vi "LinearIndicatorMarker.vi"(4 "Marker Height":i32, 5 "Group":string, 6 "Value":dbl, 7 "Color":u32(colorbox)=6618880, 10 "RectangleSizeAndLocation":T2, 11 "Image":T1) -> (3 "Image Out":T1)   [LabVIEW 2015]
uses:
  <vilib>/vision/Image Controls.llb/IMAQ Image.ctl
panel:
  in  "HorizontalOffset":i32
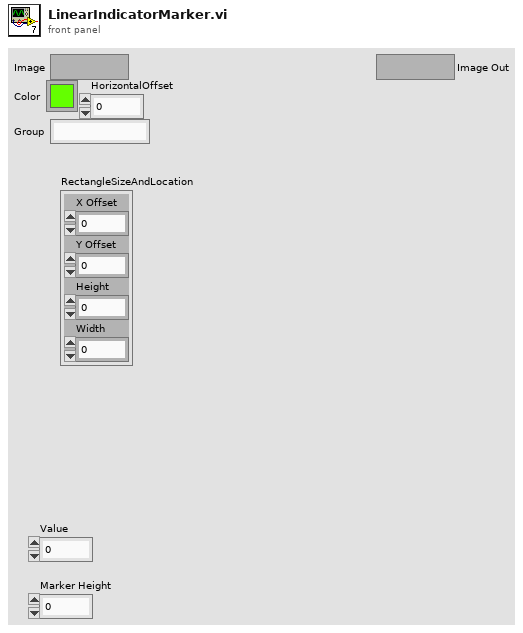
[diagram p1: front panel]
types:
  T1 = typedef "IMAQ Image.ctl" = refnum<image>
  T2 = cluster{"X Offset":i32, "Y Offset":i32, "Height":i32, "Width":i32}
  T3 = cluster{"Left":i32, "Top":i32, "Right":i32, "Bottom":i32}
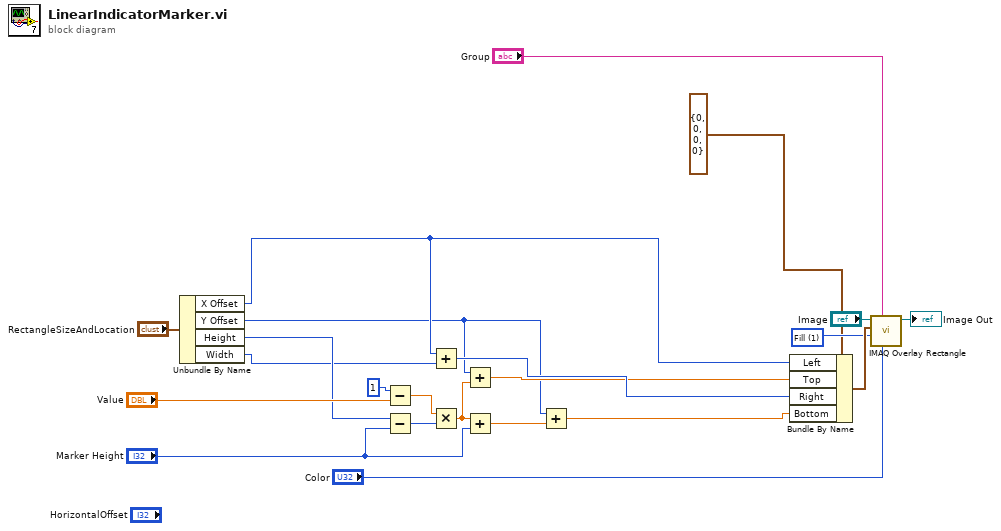
[diagram p0: block diagram]
diagram:
  w19 = u32 1 items=["Frame", "Fill", "Highlight"] ("Drawing Mode (Frame)")
  n1 = Unbundle By Name("RectangleSizeAndLocation") -> ("X Offset"=w7:i32, "Y Offset"=w6:i32, "Height"=w5:i32, "Width"=w4:i32)
  n2 = Subtract(x=1, y="Value") -> (x-y=w15:dbl)
  n3 = Subtract(x=w5, y="Marker Height") -> (x-y=w16:i32)
  n4 = Add(x=w7, y=w4) -> (x+y=w21:i32)
  n5 = Multiply(x=w15, y=w16) -> (x*y=w12:dbl)
  n6 = Add(x=w6, y=w12) -> (x+y=w10:dbl)
  n7 = Add(x=w12, y="Marker Height") -> (x+y=w13:dbl)
  n8 = Add(x=w6, y=w13) -> (x+y=w11:dbl)
  n9 = Bundle By Name(cluster=T3 {"Left"=0, "Top"=0, "Right"=0, "Bottom"=0} ("Rectangle"), "Left"=w7, "Top"=w10, "Right"=w21, "Bottom"=w11) -> (w20:T3)
  n10 = call "IMAQ Overlay Rectangle"("Color"="Color", "Group"="Group", "Drawing Mode (Frame)"=w19, "Rectangle"=w20, "Image"="Image") -> ("Image Out"=→"Image Out":T1)  [unwired: 5 in, 1 out]
